vi "_WriteSubData_TDMS_SMP.vi"(8 "error in (no error)":errorcluster, 10 "Sub Data in":T1 {"Control"."motor_ctrl_array"."sensor" format="%#.2f"; "Control"."motor_ctrl_array"."setpoint" format="%#.2f"; "Control"."dac_outputs" format="%#.2f"; "PWR"."motor_array"."motor_name" items=["Motor1", "Motor2", "Motor3", "Motor4", "Motor5", "Motor6"]}, 11 "Refnum in":refnum<k34>) -> (0 "error out":errorcluster, 3 "Refnum out":refnum<k34>)   [LabVIEW 2018]
uses:
  TypeDefsSubsea/Sub Data.ctl
  TypeDefsSubsea/Sub Status.ctl
  Shared/Type Defs/ROV States.ctl
  Shared/Type Defs/SMP.ctl
  Shared/Type Defs/PWR.ctl
  Shared/Type Defs/Motor.ctl
  Shared/Type Defs/MotorNames.ctl
  Shared/Type Defs/SmartCard.ctl
  Shared/Type Defs/Box Names.ctl
  TypeDefsSubsea/Sub Control.ctl
  TypeDefsSubsea/Modos Control.ctl
  TypeDefsSubsea/ROV Outputs.ctl
  TypeDefsSubsea/Motor Control.ctl
  TypeDefsSubsea/Type Defs Subsea.lvlib
  TypeDefsTopside/Type Defs Topside.lvlib
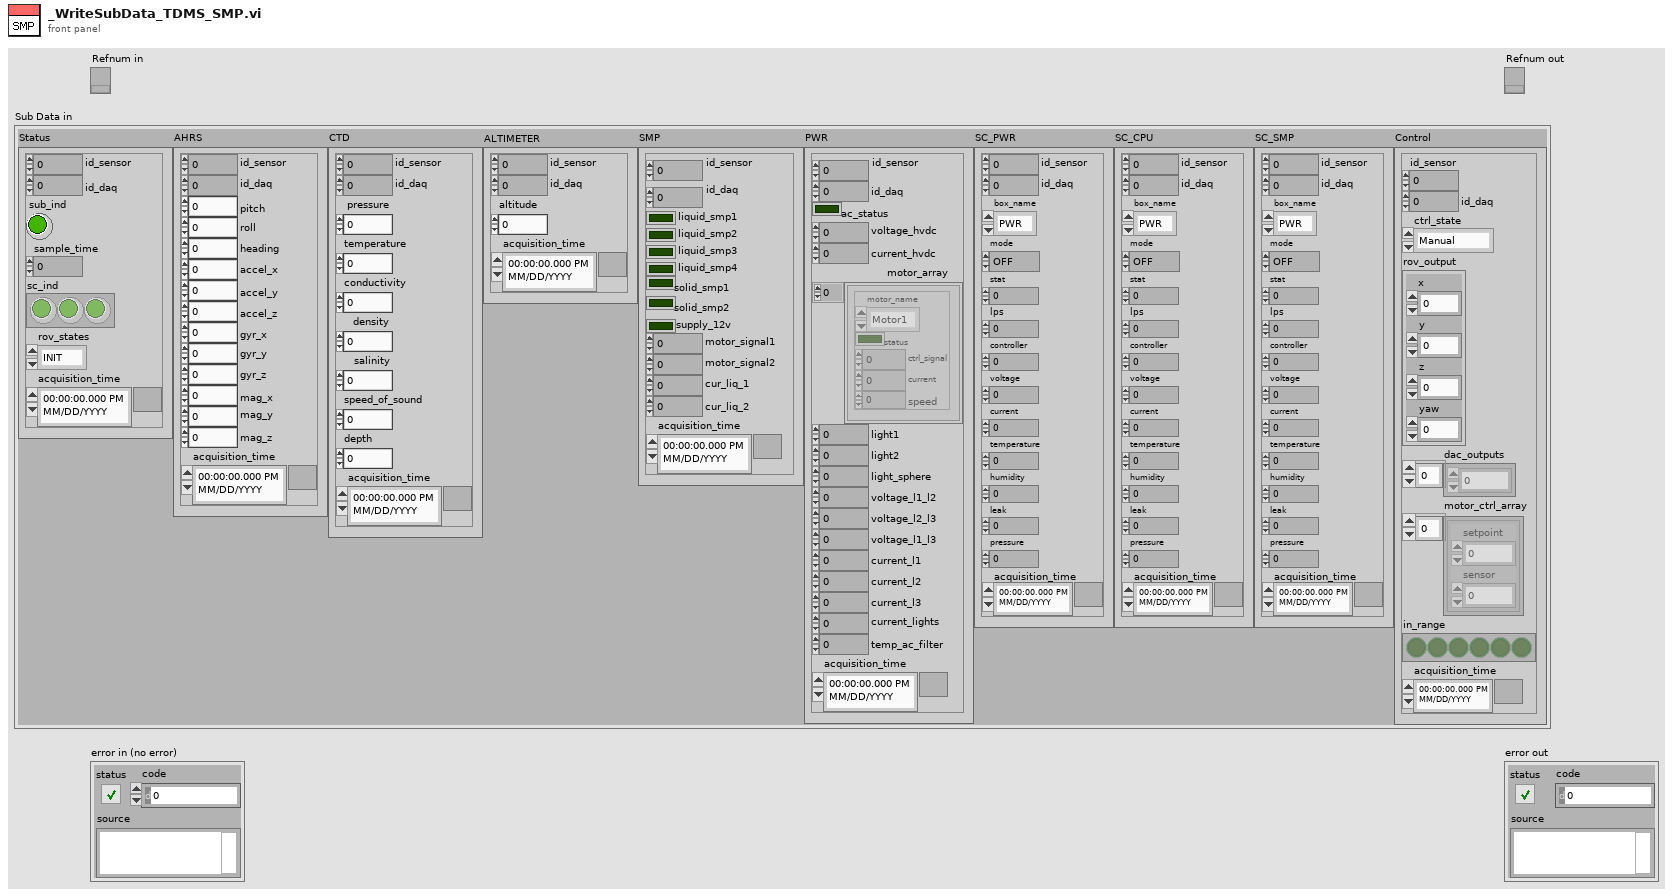
[diagram p1: front panel]
types:
  T1 = typedef "Type Defs Subsea.lvlib/Sub Data.ctl" = cluster{"Status":T2, "AHRS":cluster{"id_sensor":u32, "id_daq":u64, "pitch":dbl, "roll":dbl, "heading":dbl, "accel_x":dbl, "accel_y":dbl, "accel_z":dbl, "gyr_x":dbl, "gyr_y":dbl, "gyr_z":dbl, "mag_x":dbl, "mag_y":dbl, "mag_z":dbl, "acquisition_time":timestamp}, "CTD":cluster{"id_sensor":u32, "id_daq":u64, "pressure":dbl, "temperature":dbl, "conductivity":dbl, "density":dbl, "salinity":dbl, "speed_of_sound":dbl, "depth":dbl, "acquisition_time":timestamp}, "ALTIMETER":cluster{"id_sensor":u32, "id_daq":u64, "altitude":dbl, "acquisition_time":timestamp}, "SMP":T4, "PWR":T5, "SC_PWR":T8, "SC_CPU":T8, "SC_SMP":T8, "Control":T10}
  T2 = typedef "Type Defs Subsea.lvlib/Sub Status.ctl" = cluster{"id_sensor":u32, "id_daq":u32, "sub_ind":bool, "sample_time":i64, "sc_ind":bool[], "rov_states":T3, "acquisition_time":timestamp}
  T3 = typedef "Type Defs Subsea.lvlib/ROV States.ctl" = enum16{"INIT", "IDLE", "TEST", "RUN", "EMERGENCY", "EXIT"}
  T4 = typedef "Type Defs Subsea.lvlib/SMP.ctl" = cluster{"id_sensor":u32, "id_daq":u64, "liquid_smp1":bool, "liquid_smp2":bool, "liquid_smp3":bool, "liquid_smp4":bool, "solid_smp1":bool, "solid_smp2":bool, "supply_12v":bool, "motor_signal1":dbl, "motor_signal2":dbl, "cur_liq_1":dbl, "cur_liq_2":dbl, "acquisition_time":timestamp}
  T5 = typedef "Type Defs Topside.lvlib/PWR.ctl" = cluster{"id_sensor":u32, "id_daq":u64, "ac_status":bool, "voltage_hvdc":dbl, "current_hvdc":dbl, "motor_array":T6[], "light1":dbl, "light2":dbl, "light_sphere":dbl, "voltage_l1_l2":dbl, "voltage_l2_l3":dbl, "voltage_l1_l3":dbl, "current_l1":dbl, "current_l2":dbl, "current_l3":dbl, "current_lights":dbl, "temp_ac_filter":dbl, "acquisition_time":timestamp}
  T6 = typedef "Type Defs Subsea.lvlib/Motor.ctl" = cluster{"motor_name":T7, "status":bool, "ctrl_signal":dbl, "current":dbl, "speed":dbl}
  T7 = typedef "Type Defs Subsea.lvlib/MotorNames.ctl" = u16
  T8 = typedef "Type Defs Subsea.lvlib/SmartCard.ctl" = cluster{"id_sensor":u32, "id_daq":u64, "box_name":T9, "mode":enum16{"OFF", "STANDBY", "TESTING", "RUN", "EMERGENCY"}, "stat":dbl, "lps":dbl, "controller":dbl, "voltage":dbl, "current":dbl, "temperature":dbl, "humidity":dbl, "leak":dbl, "pressure":dbl, "acquisition_time":timestamp}
  T9 = typedef "Type Defs Subsea.lvlib/Box Names.ctl" = enum16{"PWR", "CPU", "SMP"}
  T10 = typedef "Type Defs Subsea.lvlib/Sub Control.ctl" = cluster{"id_sensor":u32, "id_daq":u64, "ctrl_state":T11, "rov_output":T12, "dac_outputs":dbl[], "motor_ctrl_array":T13[], "in_range":bool[], "acquisition_time":timestamp}
  T11 = typedef "Type Defs Subsea.lvlib/Modos Control.ctl" = enum16{"Manual", "Profundidad", "Altitud", "Rumbo", "P+R"}
  T12 = typedef "Type Defs Subsea.lvlib/ROV Outputs.ctl" = cluster{"x":dbl, "y":dbl, "z":dbl, "yaw":dbl}
  T13 = typedef "Type Defs Subsea.lvlib/Motor Control.ctl" = cluster{"setpoint":dbl, "sensor":dbl}
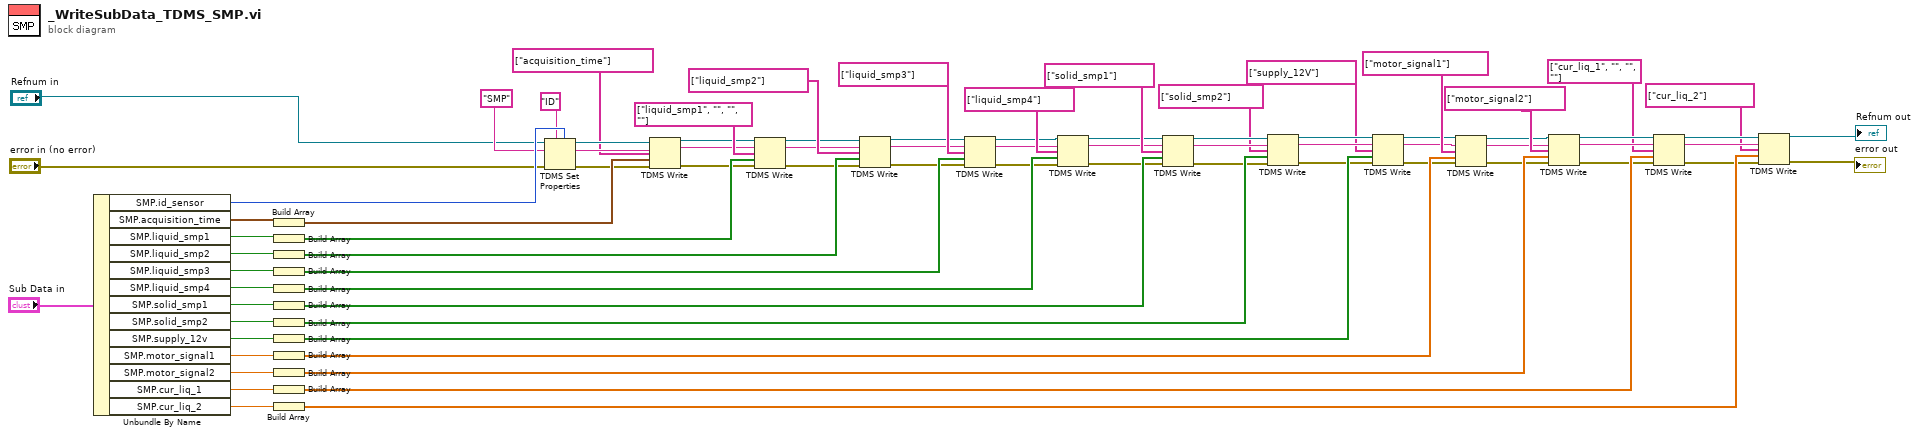
[diagram p0: block diagram]
diagram:
  n1 = Unbundle By Name("Sub Data in") -> ("SMP.id_sensor"=w63:u32, "SMP.acquisition_time"=w64:timestamp, "SMP.liquid_smp1"=w65:bool, "SMP.liquid_smp2"=w66:bool, "SMP.liquid_smp3"=w67:bool, "SMP.liquid_smp4"=w68:bool, "SMP.solid_smp1"=w9:bool, "SMP.solid_smp2"=w8:bool, "SMP.supply_12v"=w7:bool, "SMP.motor_signal1"=w6:dbl, "SMP.motor_signal2"=w5:dbl, "SMP.cur_liq_1"=w4:dbl, "SMP.cur_liq_2"=w3:dbl)
  n2 = Build Array(w64) -> (w69:timestamp[])
  n3 = Build Array(w65) -> (w70:bool[])
  n4 = Build Array(w66) -> (w71:bool[])
  n5 = Build Array(w67) -> (w72:bool[])
  n6 = Build Array(w68) -> (w73:bool[])
  n7 = Build Array(w9) -> (w74:bool[])
  n8 = Build Array(w8) -> (w75:bool[])
  n9 = Build Array(w7) -> (w76:bool[])
  n10 = Build Array(w6) -> (w77:dbl[])
  n11 = Build Array(w5) -> (w78:dbl[])
  n12 = Build Array(w4) -> (w79:dbl[])
  n13 = Build Array(w3) -> (w80:dbl[])
  n14 = TDMS Set Properties(5:w63, 7:"ID" ("property names"), 8:"error in (no error)", 10:"SMP" ("group name in (Untitled)"), 11:"Refnum in") -> (0:w22:errorcluster, 2:w21:string, 3:w19:refnum<k34>)  [unwired: 1 in, 1 out]
  n15 = TDMS Write(0:w19, 5:w21, 7:string[] ["acquisition_time"] ("channel name(s) in (Untitled)"), 9:w69, 11:w22) -> (4:w15:refnum<k34>, 6:w14:string, 15:w16:errorcluster)  [unwired: 1 in, 1 out]
  n16 = TDMS Write(0:w15, 5:w14, 7:string[] ["liquid_smp1", "", "", ""] ("channel name(s) in (Untitled)"), 9:w70, 11:w16) -> (4:w27:refnum<k34>, 6:w26:string, 15:w28:errorcluster)  [unwired: 1 in, 1 out]
  n17 = TDMS Write(0:w27, 5:w26, 7:string[] ["liquid_smp2"] ("channel name(s) in (Untitled)"), 9:w71, 11:w28) -> (4:w24:refnum<k34>, 6:w23:string, 15:w25:errorcluster)  [unwired: 1 in, 1 out]
  n18 = TDMS Write(0:w24, 5:w23, 7:string[] ["liquid_smp3"] ("channel name(s) in (Untitled)"), 9:w72, 11:w25) -> (4:w42:refnum<k34>, 6:w43:string, 15:w61:errorcluster)  [unwired: 1 in, 1 out]
  n19 = TDMS Write(0:w42, 5:w43, 7:string[] ["liquid_smp4"] ("channel name(s) in (Untitled)"), 9:w73, 11:w61) -> (4:w40:refnum<k34>, 6:w41:string, 15:w39:errorcluster)  [unwired: 1 in, 1 out]
  n20 = TDMS Write(0:w40, 5:w41, 7:string[] ["solid_smp1"] ("channel name(s) in (Untitled)"), 9:w74, 11:w39) -> (4:w34:refnum<k34>, 6:w35:string, 15:w33:errorcluster)  [unwired: 1 in, 1 out]
  n21 = TDMS Write(0:w34, 5:w35, 7:string[] ["solid_smp2"] ("channel name(s) in (Untitled)"), 9:w75, 11:w33) -> (4:w37:refnum<k34>, 6:w38:string, 15:w36:errorcluster)  [unwired: 1 in, 1 out]
  n22 = TDMS Write(0:w37, 5:w38, 7:string[] ["supply_12V"] ("channel name(s) in (Untitled)"), 9:w76, 11:w36) -> (4:w56:refnum<k34>, 6:w58:string, 15:w57:errorcluster)  [unwired: 1 in, 1 out]
  n23 = TDMS Write(0:w56, 5:w58, 7:string[] ["motor_signal1"] ("channel name(s) in (Untitled)"), 9:w77, 11:w57) -> (4:w53:refnum<k34>, 6:w54:string, 15:w59:errorcluster)  [unwired: 1 in, 1 out]
  n24 = TDMS Write(0:w53, 5:w54, 7:string[] ["motor_signal2"] ("channel name(s) in (Untitled)"), 9:w78, 11:w59) -> (4:w51:refnum<k34>, 6:w52:string, 15:w50:errorcluster)  [unwired: 1 in, 1 out]
  n25 = TDMS Write(0:w51, 5:w52, 7:string[] ["cur_liq_1", "", "", ""] ("channel name(s) in (Untitled)"), 9:w79, 11:w50) -> (4:w47:refnum<k34>, 6:w48:string, 15:w46:errorcluster)  [unwired: 1 in, 1 out]
  n26 = TDMS Write(0:w47, 5:w48, 7:string[] ["cur_liq_2"] ("channel name(s) in (Untitled)"), 9:w80, 11:w46) -> (4:→"Refnum out":refnum<k34>, 15:→"error out":errorcluster)  [unwired: 1 in, 2 out]
